vi "Publish.vi"(6 "Publish Time":timestamp, 8 "error in (no error)":errorcluster, 9 "Data to Publish":variant, 10 "Topic Name":string, 11 "Mediator in":refnum<class "IMediator.lvclass">) -> (0 "error out":errorcluster, 3 "Mediator out":refnum<class "IMediator.lvclass">)   [LabVIEW 2015, in "IMediator.lvlib" / "IMediator.lvclass"]
uses:
  IMediator.lvclass
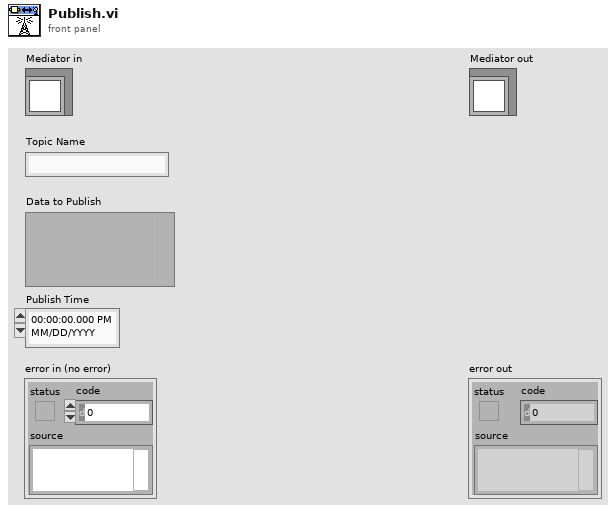
[diagram p1: front panel]
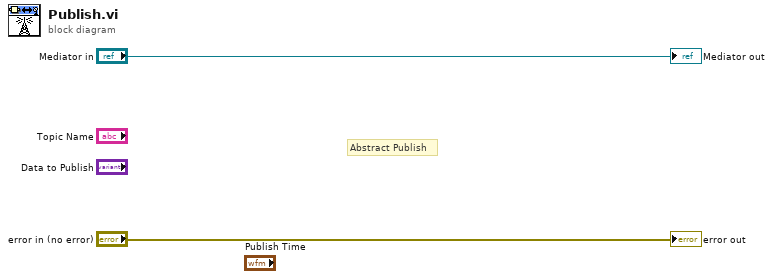
[diagram p0: block diagram]
diagram:
  # "Abstract Publish"
  "error out" <- "error in (no error)"
  "Mediator out" <- "Mediator in"
